vi "Ejercicio 4.1.vi"() -> ()   [LabVIEW 2021]
uses:
  <vilib>/ptbypt/NI_PtbyPt.lvlib
panel:
  out "Average 1":dbl
  out "Average 2":dbl
  out "Waveform Array 2":dbl[](array[numeric])
  out "Time Array, s 2":dbl[](array[numeric])
  out "Current Waveform 2":cluster{dbl[], dbl[]}(graph)
  in  "Scalar":dbl
  in  "Heigh":dbl
  in  "Phase":dbl
  in  "Time in Seconds":dbl
  in  "Sample Rate (Samples/Second)":dbl
  in  "Frecuency":dbl
  in  "Hz":dbl
  out "Time Array, s":dbl[](array[numeric])
  out "Current Waveform":cluster{dbl[], dbl[]}(graph)
  out "Waveform Array":dbl[](array[numeric])
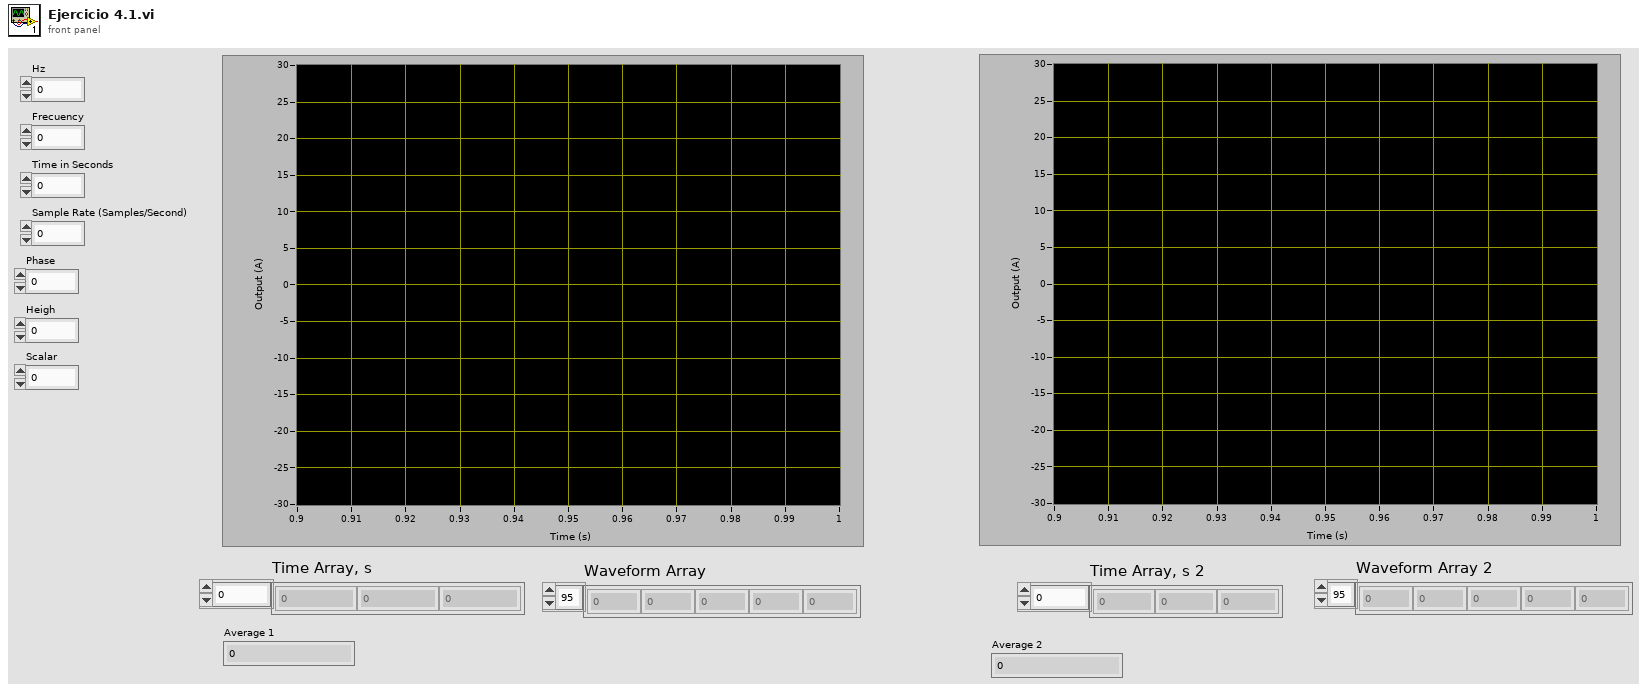
[diagram p1: front panel]
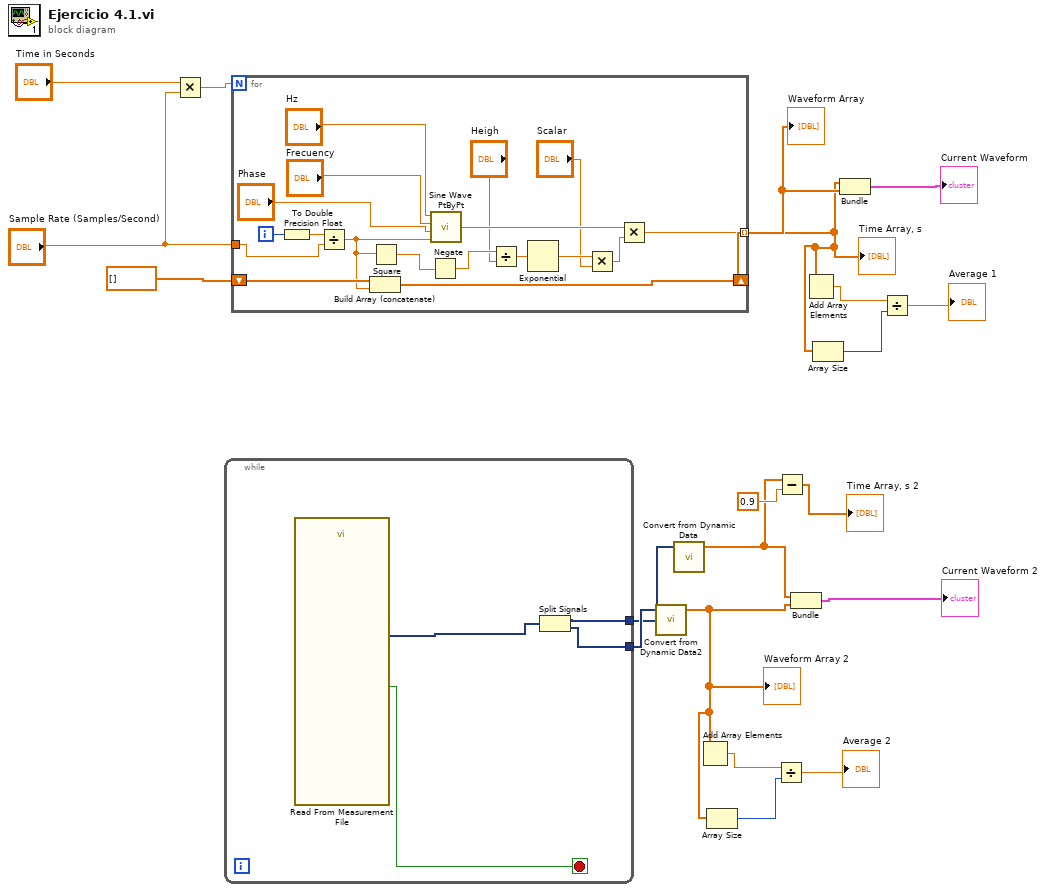
[diagram p0: block diagram]
diagram:
  n1 = Multiply(x="Time in Seconds", y="Sample Rate (Samples/Second)") -> (x*y=w15:dbl)
  n2 = while {
    tunnel: [w22] -> w12
    tunnel: [w21] -> w13
    stop <- w24 stop-if-true
    n3 = call "Read From Measurement File"() -> ("Signals"=w23:dynamicdata, "EOF?"=w24:bool)  [unwired: 6 in, 4 out]
    n4 = Split Signals(w23) -> (w22:dynamicdata, w21:dynamicdata)  [unwired: 2 in]
  }
  n5 = for {
    N: w15 -> [_]
    tunnel: "Sample Rate (Samples/Second)" -> [w28]
    tunnel: [w25] -> w16 mode=indexing
    shift-right: [w35] -> w4
    shift-left: dbl[] [] -> [w34]
    i -> [w27]
    n6 = To Double Precision Float(number=w27) -> (double precision float=w36:dbl)
    n7 = Divide(x=w36, y=w28) -> (x/y=w26:dbl)
    n8 = Build Array (concatenate)(w34, w26) -> (w35:dbl[])
    n9 = Square(x=w26) -> (x^2=w38:dbl)
    n10 = Negate(x=w38) -> (-x=w39:dbl)
    n11 = call <vilib>:"Sine Wave PtByPt.vi"("time"=w26, "phase"="Phase", "frequency"="Frecuency", "amplitude"="Hz") -> ("sine wave"=w42:dbl)
    n12 = Divide(x=w39, y="Heigh") -> (x/y=w40:dbl)
    n13 = Exponential(1:w40) -> (0:w41:dbl)
    n14 = Multiply(x=w41, y="Scalar") -> (x*y=w37:dbl)
    n15 = Multiply(x=w42, y=w37) -> (x*y=w25:dbl)
  }
  "Waveform Array" <- w16
  "Time Array, s" <- w4
  n16 = call "Convert from Dynamic Data2"("Dynamic Data Type"=w13) -> ("Array"=w9:dbl[])  [unwired: 3 in]
  "Waveform Array 2" <- w9
  n17 = call "Convert from Dynamic Data"("Dynamic Data Type"=w12) -> ("Array"=w2:dbl[])  [unwired: 3 in]
  n18 = Add Array Elements(numeric array=w9) -> (sum=w11:dbl)
  n19 = Array Size(array=w9) -> (size(s)=w8:i32)
  n20 = Divide(x=w11, y=w8) -> (x/y=→"Average 2":dbl)
  n21 = Subtract(x=w2, y=0.9) -> (x-y=→"Time Array, s 2":dbl[])
  n22 = Bundle("Array"=w2, "Array"=w9) -> (→"Current Waveform 2":cluster{"Array":dbl[], "Array":dbl[]})  [unwired: 1 in]
  n23 = Add Array Elements(numeric array=w4) -> (sum=w7:dbl)
  n24 = Array Size(array=w4) -> (size(s)=w5:i32)
  n25 = Bundle(w4, w16) -> (→"Current Waveform":cluster{dbl[], dbl[]})  [unwired: 1 in]
  n26 = Divide(x=w7, y=w5) -> (x/y=→"Average 1":dbl)
